vi "Main VI.vi"(10 "Numeric":dbl) -> ()   [LabVIEW 2021]
uses:
  <vilib>/measure/NI_MABase.lvlib
panel:
  out "Waveform Chart":waveform(dbl)(graph)
  out "Loop":i32
  in  "stop":bool
  out "error out":errorcluster
  in  "error in (no error)":errorcluster
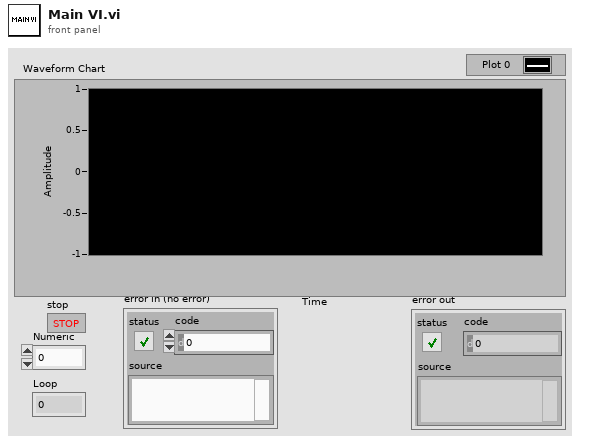
[diagram p1: front panel]
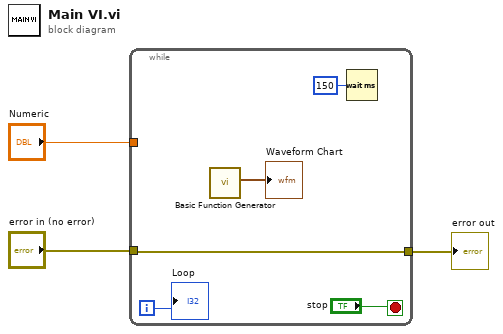
[diagram p0: block diagram]
diagram:
  n1 = while {
    tunnel: "Numeric" -> [_]
    tunnel: "error in (no error)" -> [w4]
    tunnel: [w4] -> w1
    i -> [w7]
    stop <- "stop" stop-if-true
    n2 = call <vilib>:"Basic Function Generator.vi"() -> ("signal out"=→"Waveform Chart":waveform(dbl))  [unwired: 9 in, 2 out]
    n3 = Wait (ms)(milliseconds to wait=u32 150) -> ()  [unwired: 1 out]
    "Loop" <- w7
  }
  "error out" <- w1
